vi "MS_Global.vi"() -> ()   [LabVIEW 2020]
uses:
  Controls/Idle_Timer.ctl
  Controls/Idle_Timer_disp.ctl
  Controls/PKYK_Status_Enum.ctl
  Controls/WIP Limit.ctl
  Controls/WIP_old.ctl
  Controls/WIP_ref.ctl
  Controls/TS_Parameter_V2.ctl
panel:
  out "init":bool
  in  "Slno":i32 format="%04d"
  out "DATA EXISTS":bool
  in  "Mfgr Date":timestamp
  in  "Shift":string="192.168.4.180,1,0"
  out "Traceability":bool
  out "PokaYoke ?":bool
  out "PokaYoke On?":bool
  in  "WIP Chk":i64[](array[numeric])
  out "WIP MC No":string[](array[string])=["", "OP10", "OP20", "OP30", "OP40", "OP50", "OP60", "OP70", "OP80"]
  out "TAG_CHANGE":bool[](array[boolean])
  out "Cycle_Run":bool[](array[boolean])
  out "TS Parameter":T1={"ProfitCenterCode"="", "LineCode"="", "WorkOrderNumber"="", "Model"="", "Model_with_Prefix"="", "VendorCode"="", "SetParameterDateCode"="", "PokaYoke"=0, "Target"=1, "Live_DateCode"="", "CustomerPartNumber"="", "Hose_Type"="", "sBarcode"=FALSE, "FCA"=0, "Ent_Stamp"=timestamp(0 s since 1904-01-01), "STS_CD"=0.0} {"FCA" format="%01d"; "Target" min=1 max=100000; "PokaYoke" min=0 max=1}
  out "Tag Presence":bool[](array[boolean])
  out "Machine No":string[](array[string])=["TS_CODE_OP_00", "TS_CODE_OP_10", "TS_CODE_OP_20", "TS_CODE_OP_30", "TS_CODE_OP_40", "TS_CODE_OP_50", "TS_CODE_OP_60", "TS_CODE_OP_70", "TS_CODE_OP_80", "TS_CODE_OP_90"]
  out "TS_DATA_SAVED":string[](array[string])=["TS_CODE_OP_00", "TS_CODE_OP_10", "TS_CODE_OP_20", "TS_CODE_OP_30", "TS_CODE_OP_40", "TS_CODE_OP_50", "TS_CODE_OP_60", "TS_CODE_OP_70", "TS_CODE_OP_80", "TS_CODE_OP_90"]
  out "Part Routing":bool[](array[boolean])
  out "Line Routing":bool[](array[boolean])
  out "Routing":bool[](array[boolean])
  out "Pokeyoke":bool[](array[boolean])
  out "OP Table List":string[](array[string])=["[DBO].[OP10_CRIMP]", "[DBO].[OP20_TEST_STN]", "[DBO].[OP30_VERIFY_STN]"]
  in  "TRACE_PLC_IP":string="192.168.4.180,1,0"
  in  "Bckup_DB?":bool
  in  "Pass_Timeout":dbl
  out "WIP Ref":T2
  out "WIP Limit":T3
  in  "PKYK_Status":T5
  out "PKYK_RFID?":bool
  in  "BDR_Remarks":string="Idle Time!\rEnter Breakdown/Bookout Loss"
  in  "Idle Timer":T6={"OP10"=0.2, "OP20"=0.2, "OP30"=0.2, "OP40"=0.2, "OP50"=0.2, "OP60"=0.2} {"OP60" min=0.1 max=9999999.0; "OP50" min=0.1 max=9999999.0; "OP40" min=0.1 max=9999999.0; "OP30" min=0.1 max=9999999.0; "OP20" min=0.1 max=9999999.0; "OP10" min=0.1 max=9999999.0}
  in  "Mind IP":string="USE cell10"
  out "TS_CODE_TAG":string[](array[string])=["", "OP10_TS_CODE", "OP20_TS_CODE", "OP30A_TS_CODE", "OP40_TS_CODE", "OP50_TS_CODE", "OP60_TS_CODE", "OP70_TS_CODE", "OP80_TS_CODE"]
  in  "Ent_Stamp":timestamp
  out "Part Pokeyoke":bool[](array[boolean])
  out "Line Pokeyoke":bool[](array[boolean])
  out "MachineCode":string[](array[string])=["MCIG", "MCSC", "MCCT", "MCPA", "MCLP", "MCHP", "MCFA", "MCSR", "MCDC", "MCFV"]
  out "OperationCode":string[](array[string])
  in  "Database":string="USE cell10"
  # "Idle Timer"
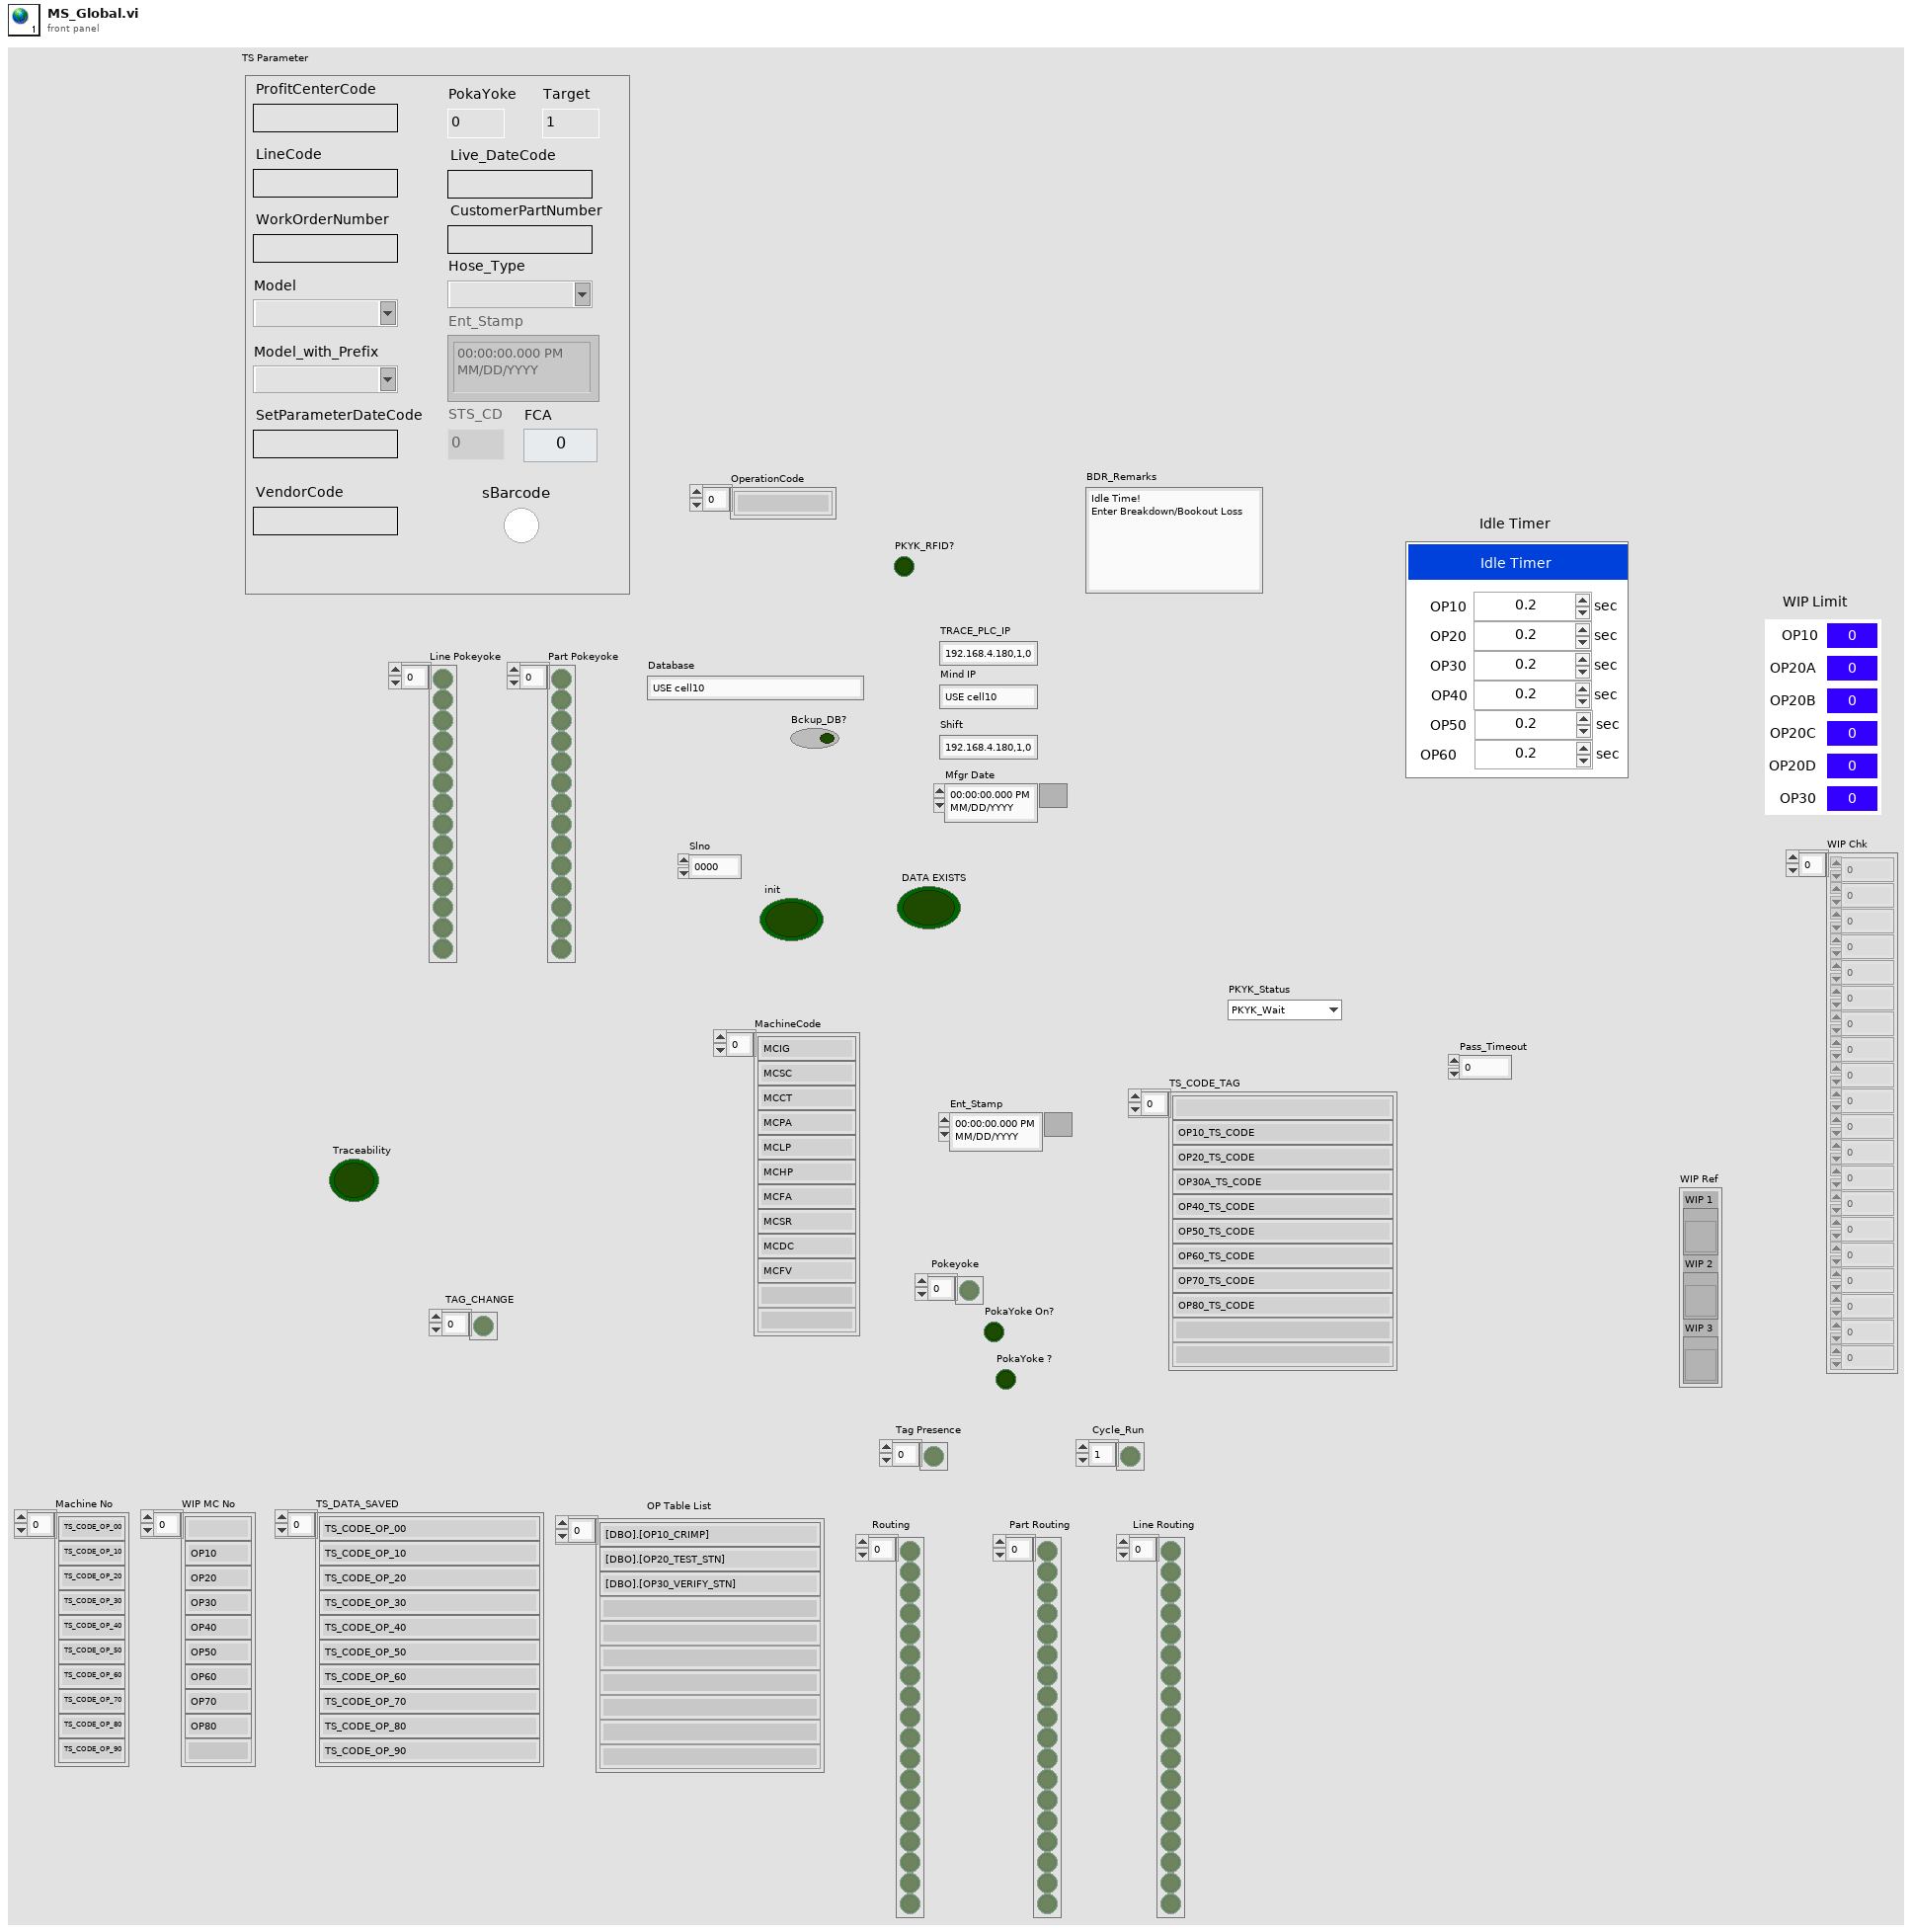
[diagram p1: front panel]
types:
  T1 = typedef "TS_Parameter_V2.ctl" = cluster{"ProfitCenterCode":string, "LineCode":string, "WorkOrderNumber":string, "Model":string, "Model_with_Prefix":string, "VendorCode":string, "SetParameterDateCode":string, "PokaYoke":i32, "Target":i32, "Live_DateCode":string, "CustomerPartNumber":string, "Hose_Type":string, "sBarcode":bool, "FCA":i32, "Ent_Stamp":timestamp, "STS_CD":dbl}
  T2 = typedef "WIP_ref.ctl" = cluster{"WIP 1":refnum<vi>, "WIP 2":refnum<vi>, "WIP 3":refnum<vi>}
  T3 = typedef "WIP Limit.ctl" = cluster{"OP10":T4, "OP20A":T4, "OP20B":T4, "OP20C":T4, "OP20D":T4, "OP30":T4}
  T4 = typedef "WIP_old.ctl" = i64
  T5 = typedef "PKYK_Status_Enum.ctl" = enum16{"PKYK_Wait", "PKYK_Done"}
  T6 = typedef "Idle_Timer.ctl" = cluster{"OP10":T7, "OP20":T7, "OP30":T7, "OP40":T7, "OP50":T7, "OP60":T7}
  T7 = typedef "Idle_Timer_disp.ctl" = dbl
diagram:
